vi "Digital Write Square Wave.vi"(7 "Duration (ms)":u32, 8 "Error In":errorcluster, 9 "Frequency (Hz)":u32, 10 "Channel":u8, 11 "LINX Resource":T1) -> (0 "Error Out":errorcluster, 3 "LINX Resource":T1)   [LabVIEW 2020, in "LMH-LINX.lvlib"]
doc: "Generate a square wave with the specified frequency for the specified duration. myRIO uses PWM channels for this function while most other devices use a DO channels.\n\nUse a duration of 0 to generate output indefinatly.\n\nUse a frequency of 0 to stop generating output."
uses:
  LMH-LINX.lvlib
  Private/Type Defs/Peripheral.ctl
  Private/Type Defs/Error Type.ctl
  Private/Device/Device.lvlib
  Private/Type Defs/Platform.ctl
  Private/Type Defs/Interface.ctl
  Private/Type Defs/LINX Ref.ctl
  Private/Device/Type Defs/Channels.ctl
  Private/Device/Type Defs/TCP Config.ctl
  Private/Device/Type Defs/LINX Device Config.ctl
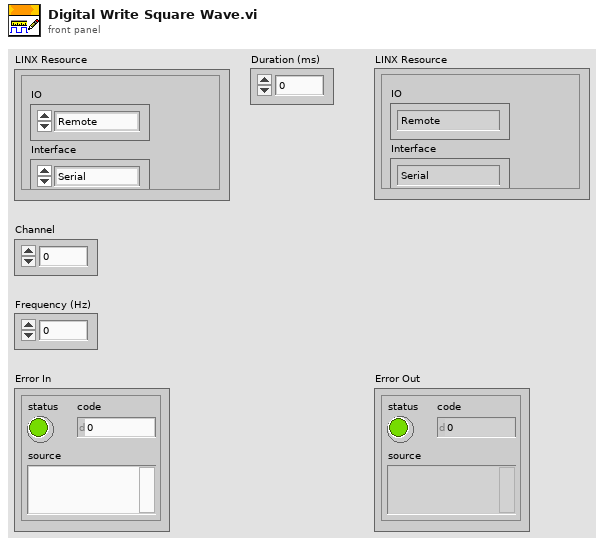
[diagram p1: front panel]
types:
  T1 = typedef "LMH-LINX.lvlib/LINX Ref.ctl" = cluster{"IO":T2, "Interface":T3, "LINX Device Config":T4}
  T2 = typedef "LMH-LINX.lvlib/Platform.ctl" = enum16{"Remote", "Local"}
  T3 = typedef "LMH-LINX.lvlib/Interface.ctl" = enum16{"Serial", "TCP"}
  T4 = typedef "Device.lvlib/LINX Device Config.ctl" = cluster{"Interface":T3, "COM Port":refnum<visa-resource-name>, "TCP Configuration":T5, "Device Family":u8, "Device ID":u8, "Device Name":string, "TCP Ref":refnum<k5>, "Channels":T6}
  T5 = typedef "Device.lvlib/TCP Config.ctl" = cluster{"IP Address":string, "Port":u16}
  T6 = typedef "LMH-LINX.lvlib/Channels.ctl" = cluster{"DI":u8[], "DO":u8[], "AI":u8[], "AO":u8[], "PWM":u8[], "QE":u8[], "UART":u8[], "I2C 2":u8[], "SPI":u8[], "CAN":u8[], "Servo":u8[], "AI Ref (V)":dbl, "AI Resolution (Bits)":u8, "AO Ref (V)":dbl, "AO Resolution (Bits)":u8}
  T7 = typedef "LMH-LINX.lvlib/Peripheral.ctl" = enum8{"DI", "DO", "AI", "AO", "PWM", "QE", "UART", "I2C", "SPI", "CAN", "Servo"}
  T8 = typedef "LMH-LINX.lvlib/Error Type.ctl" = enum16{"Unknown", "Timeout", "Corrupt Return Packet", "Unable To Connect", "Command Not Supported", "Channel DNE", "Invalid COM Config", "Firmware Version Mismatch", "myRIO Support", "CMD Specific Error", "Local IO Not Supported"}
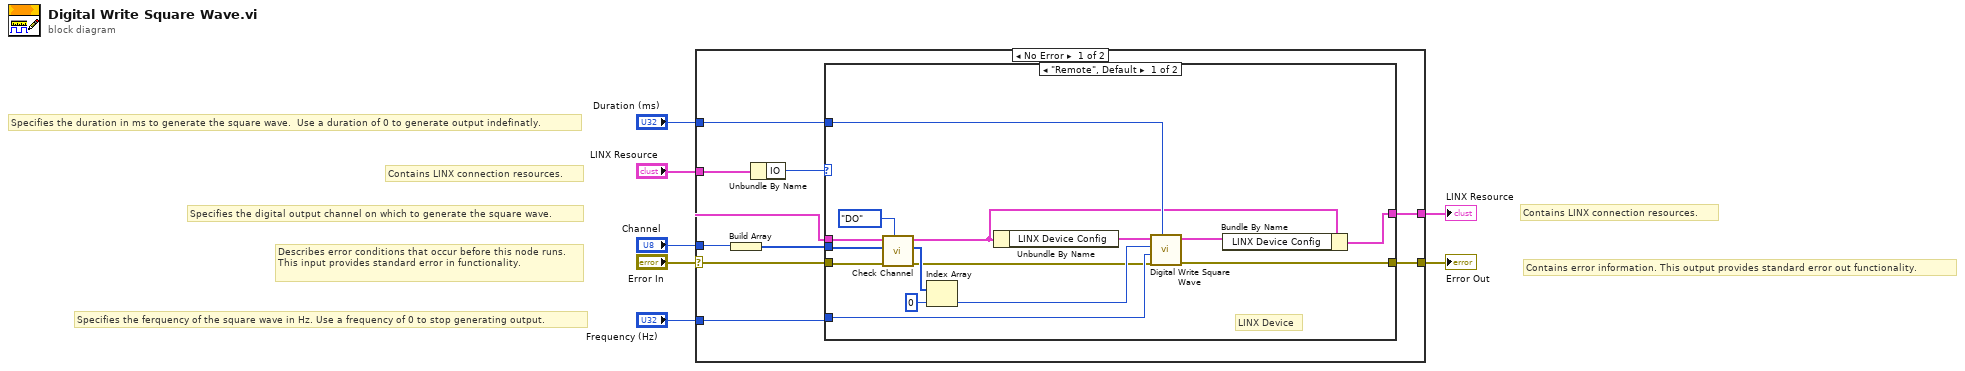
[diagram p0: block diagram]
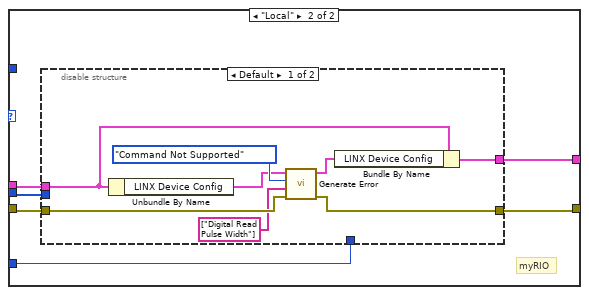
[diagram p2: hidden frame]
diagram:
  # "Specifies the ferquency of the square wave in Hz. Use a frequency of 0 to stop generating output."
  # "Specifies the digital output channel on which to generate the square wave."
  # "Specifies the duration in ms to generate the square wave.  Use a duration of 0 to generate output indefinatly."
  # "Contains LINX connection resources."
  # "Contains error information. This output provides standard error out functionality."
  # "Contains LINX connection resources."
  # "Describes error conditions that occur before this node runs. This input provides standard error in functionality."
  n1 = case shown="No Error" "Error In" {
    selector: "Error In" -> [w8 w49]
    tunnel: [w15 w49] -> w7
    tunnel: [w14 w48] -> w6
    tunnel: "Channel" -> [w13 _]
    tunnel: "Duration (ms)" -> [w12 _]
    tunnel: "Frequency (Hz)" -> [w11 _]
    tunnel: "LINX Resource" -> [w9 w48]
    frame No Error {
      n2 = Build Array(w13) -> (w10:u8[])
      n3 = Unbundle By Name(w9) -> ("IO"=w16:T2)
      n4 = case shown="\"Remote\", Default" w16 {
        tunnel: w8 -> [w23 w37]
        tunnel: w9 -> [w20 w36]
        tunnel: [w27 w32] -> w15
        tunnel: [w31 w34] -> w14
        tunnel: w10 -> [w18 w35]
        tunnel: w12 -> [w24 _]
        tunnel: w11 -> [w25 w33]
        frame "Remote", Default {
          # "LINX Device"
          n5 = call "Check Channel.vi"("Peripheral"=Peripheral."DO", "Error In"=w23, "Channels"=w18, "LINX Resource"=w20) -> ("Error Out"=w21:errorcluster, "Channels"=w22:u8[], "LINX Resource"=w19:T1)  [unwired: 5 in]
          n6 = Index Array(array=w22, index=0) -> (element=w26:u8)
          n7 = Unbundle By Name(w19) -> ("LINX Device Config"=w29:T4)
          n8 = call "Digital Write Square Wave.vi"("Duration (ms)"=w24, "Error In"=w21, "Frequency"=w25, "DO Channel"=w26, "LINX Device Config"=w29) -> ("Error Out"=w27:errorcluster, "LINX Device Config"=w28:T4)  [unwired: 5 in]
          n9 = Bundle By Name(cluster=w19, "LINX Device Config"=w28) -> (w31:T1)
        }
        frame "Local" {
          # "myRIO"
          n10 = disable-structure shown="Default" {
            disable-tunnel: w37 -> [w41 w47]
            disable-tunnel: w36 -> [w42 w46]
            disable-tunnel: w35 -> [_ _]
            disable-tunnel: [w38 w46] -> w34
            disable-tunnel: w33 -> [_ _]
            disable-tunnel: [w40 w47] -> w32
            frame condition #0 (active) {
              n11 = Unbundle By Name(w42) -> ("LINX Device Config"=w44:T4)
              n12 = call "Generate Error.vi"("Error In"=w41, "Arguments"=string[] ["Digital Read Pulse Width"], "Error Type"=Error_Type."Command Not Supported", "LINX Device Config"=w44) -> ("Error Out"=w40:errorcluster, "Dup LINX Device Config"=w43:T4)  [unwired: 6 in]
              n13 = Bundle By Name(cluster=w42, "LINX Device Config"=w43) -> (w38:T1)
            }
            frame condition #1 {
            }
          }
        }
      }
    }
    frame Error {
    }
  }
  "Error Out" <- w7
  "LINX Resource" <- w6
